vi "HART.vi"(4 "Error In":errorcluster, 7 "Command":string) -> (0 "Error Out":errorcluster, 3 "Response":string)   [LabVIEW 2018]
uses:
  MOKO_LabViewLibrary/MokoLowLevel/MokoLowLovelControl/MLLC_ConnectCluster.ctl
  MOKO_LabViewLibrary/MokoLowLevel/MokoLowLovelControl/MLLC_InterfaceType.ctl
  MOKO_LabViewLibrary/MokoLowLevel/MokoLowLovelControl/MLLC_OpenedSession.ctl
  MOKO_LabViewLibrary/MokoLowLevel/MokoLowLovelControl/MLLC_InterfaceSettings.ctl
  MOKO_LabViewLibrary/MokoLowLevel/MokoLowLovelControl/MLLC_InterfaceKind.ctl
panel:
  in  "Settings":T6={"Saved Data"=variant, "Permanent data"={"Connect"={"InterfaceType"=enum."VISA", "OpenedSession"="", "InterfaceSettings"={"Interface"=enum."RS232", "EOS 4 read"=enum."LF (\\n)", "EOS 4 write"=enum."LF (\\n)", "TMO, ms"=10000, "Sett"=variant(cluster{"Baud Rate":u32, "Data Bits":u16, "Parity":u16, "Stop Bits":u16, "Flow Control":u16, "Eho":bool} {"Baud Rate"=75, "Data Bits"=0, "Parity"=0, "Stop Bits"=0, "Flow Control"=0, "Eho"=FALSE})}}, "Value"={"I"=0.0, "P"=0.0, "T"=0.0}, "String"="empty"}}
  in  "Error Code":u32
  in  "Driver Name":string="HART"
  in  "Mode":T7(ring)=enum."Check"
  # "HART"
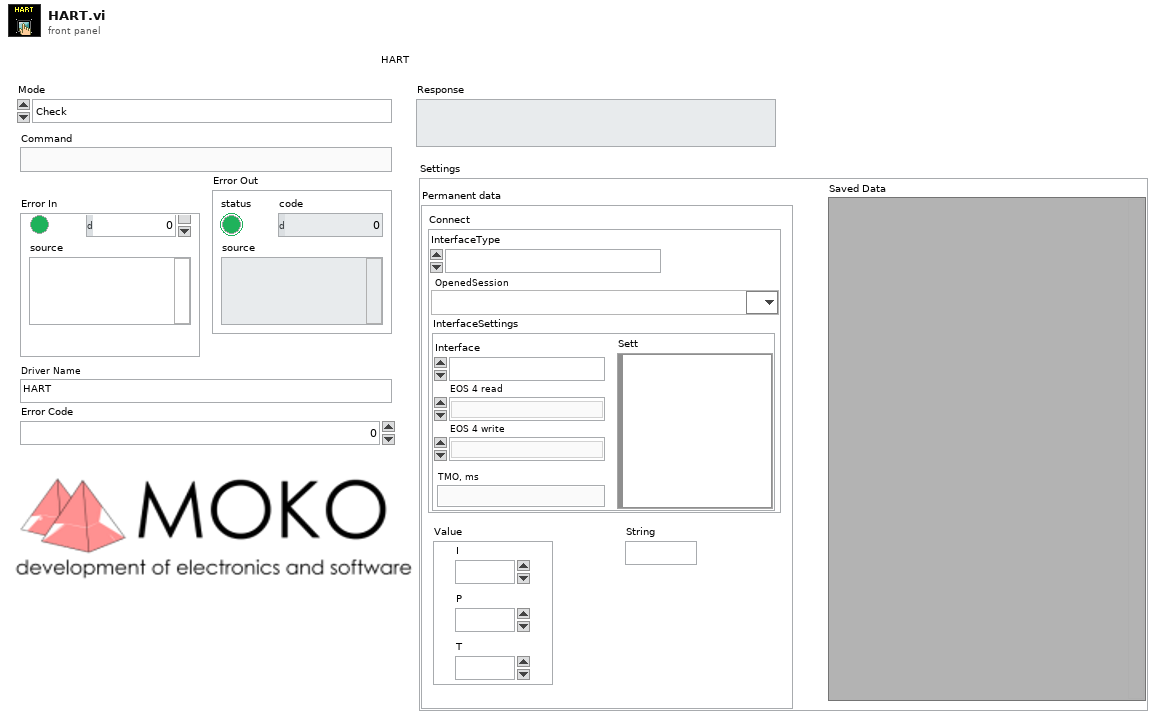
[diagram p1: front panel]
types:
  T1 = typedef "MLLC_ConnectCluster.ctl" = cluster{"InterfaceType":T2, "OpenedSession":T3, "InterfaceSettings":T4}
  T2 = typedef "MLLC_InterfaceType.ctl" = enum16{"VISA", "Prologix USB-GPIB"}
  T3 = typedef "MLLC_OpenedSession.ctl" = refnum<visa-resource-name>
  T4 = typedef "MLLC_InterfaceSettings.ctl" = cluster{"Interface":T5, "EOS 4 read":enum16{"Default (=EOS 4 write)", "CR (\\r)", "LF (\\n)", "None"}, "EOS 4 write":enum16{"CR+LF (\\r\\n)", "CR (\\r)", "LF (\\n)", "None"}, "TMO, ms":i32, "Sett":variant}
  T5 = typedef "MLLC_InterfaceKind.ctl" = enum16{"RS232", "GPIB", "USB", "Ethernet", "another"}
  T6 = cluster{"Saved Data":variant, "Permanent data":cluster{"Connect":T1, "Value":cluster{"I":dbl, "P":dbl, "T":dbl}, "String":string}}
  T7 = enum16{"get", "set", "close", "Init", "Check", "ID"}
  T8 = cluster{"Connect":T1, "Value":cluster{"I":dbl, "P":dbl, "T":dbl}, "String":string}
  T9 = typedef "MLLC_Mode.ctl" = enum16{"get", "set", "close", "Init", "Check"}
  T10 = typedef "MLLC_Error.ctl" = errorcluster
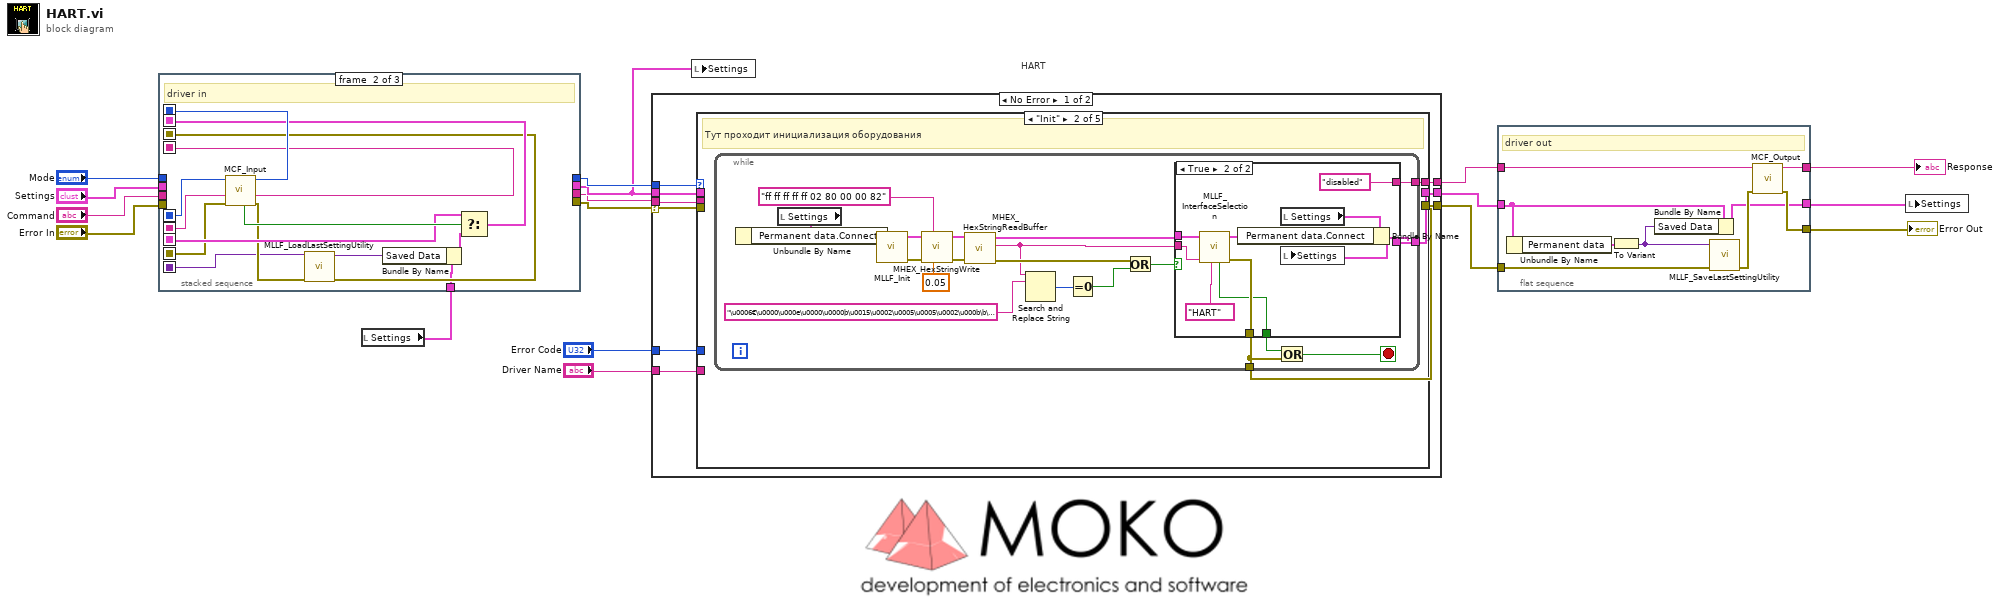
[diagram p0: block diagram]
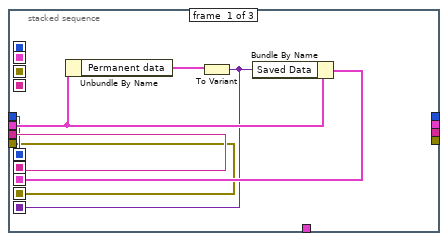
[diagram p2: hidden frame]
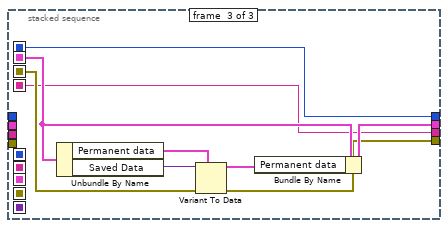
[diagram p3: hidden frame]
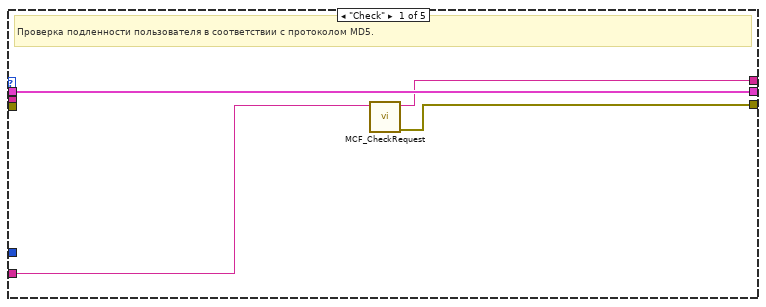
[diagram p4: hidden frame]
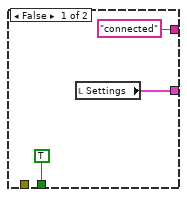
[diagram p5: hidden frame]
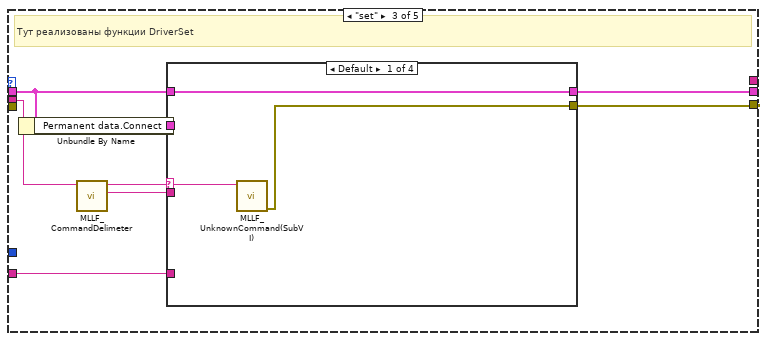
[diagram p6: hidden frame]
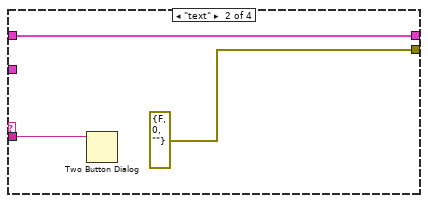
[diagram p7: hidden frame]
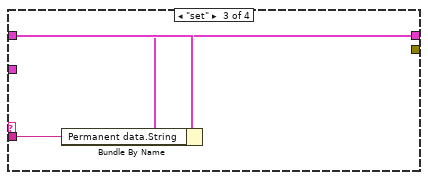
[diagram p8: hidden frame]
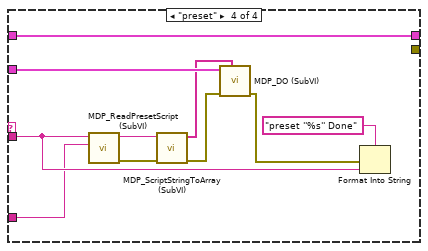
[diagram p9: hidden frame]
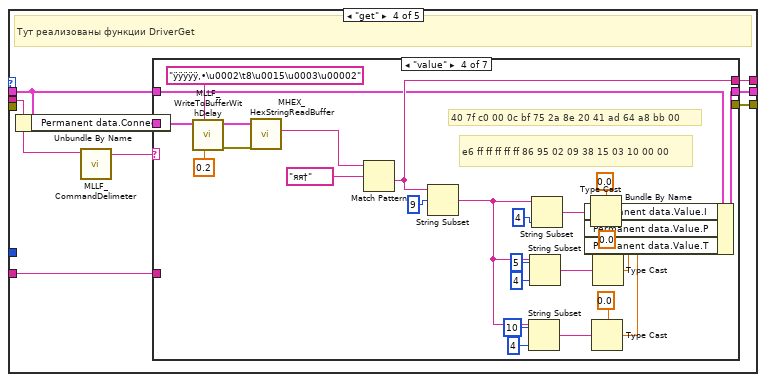
[diagram p10: hidden frame]
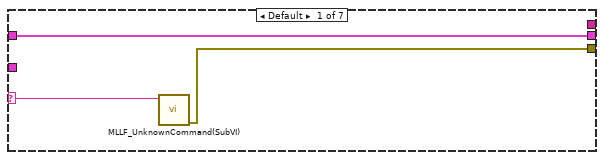
[diagram p11: hidden frame]
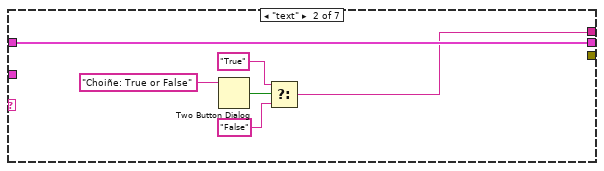
[diagram p12: hidden frame]
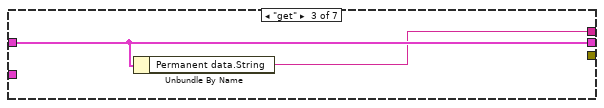
[diagram p13: hidden frame]
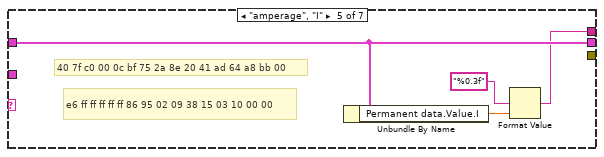
[diagram p14: hidden frame]
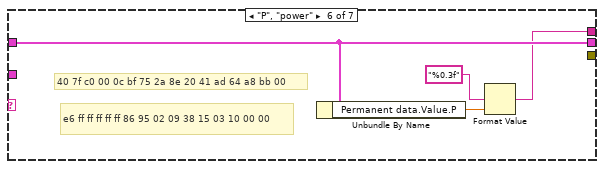
[diagram p15: hidden frame]
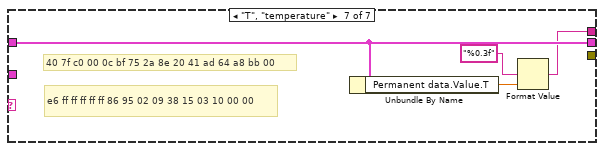
[diagram p16: hidden frame]
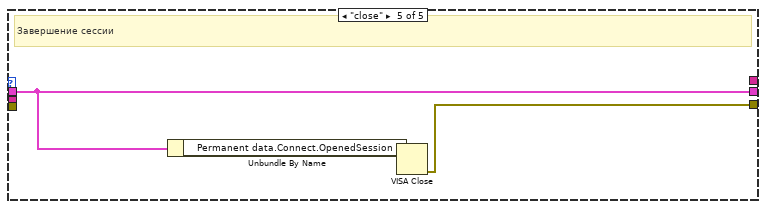
[diagram p17: hidden frame]
diagram:
  # "HART"
  n1 = local read "Settings"() -> (w13:T6)
  n2 = stacked-sequence {
    seq-local: [w20 _ _] -> [_ w36 _]
    seq-local: [w19 _ _] -> [_ w37 _]
    seq-local: [w22 _ _] -> [_ w32 _]
    seq-local: [w18 _ _] -> [_ w31 _]
    seq-local: [w21 _ _] -> [_ w27 _]
    seq-local: [_ w28 _] -> [_ _ w44]
    seq-local: [_ w38 _] -> [_ _ w41]
    seq-local: [_ w35 _] -> [_ _ w40]
    seq-local: [_ w34 _] -> [_ _ w45]
    tunnel: "Command" -> [w20 _ _]
    tunnel: "Mode" -> [w19 _ _]
    tunnel: "Error In" -> [w18 _ _]
    tunnel: "Settings" -> [w23 _ _]
    tunnel: w13 -> [_ w26 _]
    tunnel: [_ _ w40] -> w12
    tunnel: [_ _ w43] -> w14
    tunnel: [_ _ w42] -> w11
    tunnel: [_ _ w41] -> w15
    frame #0 {
      n3 = Unbundle By Name(w23) -> ("Permanent data"=w24:T8)
      n4 = To Variant(anything=w24) -> (Variant=w21:variant)
      n5 = Bundle By Name(cluster=w23, "Saved Data"=w21) -> (w22:T6)
    }
    frame #1 {
      # "driver in"
      n6 = call "MCF_Input.vi"("Error In"=w31, "Command in"=w36, "Mode in"=w37) -> ("Error Out"=w30:errorcluster, "Command out"=w35:string, "Mode out"=w38:T9, "Boolean"=w33:bool)  [unwired: 5 in]
      n7 = call "MLLF_LoadLastSettingUtility.vi"("Error In"=w30, "Save data in"=w27) -> ("Error Out"=w28:errorcluster, "Save data out"=w25:variant)  [unwired: 8 in]
      n8 = Bundle By Name(cluster=w26, "Saved Data"=w25) -> (w29:T6)
      n9 = Select(t=w32, s=w33, f=w29) -> (s? t:f=w34:T6)
    }
    frame #2 {
      n10 = Unbundle By Name(w45) -> ("Permanent data"=w46:T8, "Saved Data"=w39:variant)
      n11 = Variant To Data(error in=w44, type=w46, Variant=w39) -> (data=w47:T8, error out=w42:errorcluster)
      n12 = Bundle By Name(cluster=w45, "Permanent data"=w47) -> (w43:T6)
    }
  }
  n13 = case shown="No Error" w11 {
    selector: w11 -> [w53 w184]
    tunnel: [w48 w184] -> w4
    tunnel: w15 -> [w56 _]
    tunnel: [w55 _] -> w6
    tunnel: w12 -> [w54 _]
    tunnel: w14 -> [w50 w183]
    tunnel: "Error Code" -> [w52 _]
    tunnel: "Driver Name" -> [w51 _]
    tunnel: [w49 w183] -> w5
    frame No Error {
      n14 = case shown="\"Init\"" w56 {
        tunnel: [w58 w62 _ w124 _] -> w55
        tunnel: w54 -> [_ _ w99 w127 _]
        tunnel: w53 -> [_ _ _ _ _]
        tunnel: w52 -> [_ _ _ _ _]
        tunnel: w51 -> [w59 _ w101 w125 _]
        tunnel: w50 -> [w60 _ w103 w130 w181]
        tunnel: [w60 w63 w102 w129 w181] -> w49
        tunnel: [w57 w61 w96 w123 w180] -> w48
        frame "Check" {
          # "Проверка подленности пользователя в соответствии с протоколом MD5."
          n15 = call "MCF_CheckRequest.vi"("Driver Name"=w59) -> ("Error Out"=w57:errorcluster, "Output String"=w58:string)  [unwired: 9 in]
        }
        frame "Init" {
          # "Тут проходит инициализация оборудования"
          n16 = while {
            tunnel: [w80] -> w63
            tunnel: [w78] -> w62
            tunnel: [w65] -> w61
            stop <- w82 stop-if-true
            n17 = local read "Settings"() -> (w81:T6)
            n18 = Unbundle By Name(w81) -> ("Permanent data.Connect"=w79:T1)
            n19 = call "MLLF_Init.vi"("DriverConnect in"=w79) -> ("Error Out"=w75:errorcluster, "DriverConnect out"=w76:T1)  [unwired: 7 in]
            n20 = call "MHEX_HexStringWrite.vi"("Delay Time (s)"=0.05, "Command"="ff ff ff ff ff 02 80 00 00 82" ("commands"), "error in"=w75, "DriverConnect in"=w76) -> ("error out"=w73:T10, "DriverConnect out"=w74:T1)  [unwired: 6 in]
            n21 = call "MHEX_HexStringReadBuffer.vi"("error in"=w73, "DriverConnect in"=w74) -> ("error out"=w68:T10, "String from device out"=w64:string, "DriverConnect out"=w72:T1)  [unwired: 6 in, 1 out]
            n22 = Search and Replace String(input string=w64, search string="\u0006€\u0000\u000e\u0000\u0000þ\u0015\u0002\u0005\u0005\u0002\u000b\b\u0000\t8\u0015D\u0000") -> (number of replacements=w70:i32)  [unwired: 6 in, 3 out]
            n23 = Equal To 0?(x=w70) -> (x = 0?=w69:bool)
            n24 = Or(x=w68, y=w69) -> (x .or. y?=w67:bool)
            n25 = case shown="True" w67 {
              tunnel: w72 -> [_ w94]
              tunnel: [TRUE w89] -> w83
              tunnel: [_ w95] -> w65
              tunnel: [w85 w90] -> w80
              tunnel: ["connected" "disabled"] -> w78
              tunnel: w64 -> [_ w87]
              frame False {
                n26 = local read "Settings"() -> (w85:T6)
              }
              frame True {
                n27 = call "MLLF_InterfaceSelection.vi"("Driver Name"="HART" ("String"), "Answer:"=w87, "DriverConnect in"=w94) -> ("error out"=w95:T10, "DriverConnect out"=w92:T1, "stop init?"=w89:bool)  [unwired: 4 in, 2 out]
                n28 = local read "Settings"() -> (w91:T6)
                n29 = Bundle By Name(cluster=w91, "Permanent data.Connect"=w92) -> (w90:T6)
                n30 = local write "Settings"(w90) -> ()
              }
            }
            n31 = Or(x=w83, y=w65) -> (x .or. y?=w82:bool)
          }
        }
        frame "set" {
          # "Тут реализованы функции DriverSet"
          n32 = Unbundle By Name(w103) -> ("Permanent data.Connect"=w100:T1)
          n33 = call "MLLF_CommandDelimeter.vi"("command with param"=w99) -> ("param 1"=w97:string, "command"=w98:string)  [unwired: 6 in, 3 out]
          n34 = case shown="Default" w98 {
            selector: w98 -> [w105 _ _ _]
            tunnel: [w106 w109 w111 w113] -> w102
            tunnel: w103 -> [w106 w109 w112 w113]
            tunnel: w100 -> [_ _ _ w117]
            tunnel: w97 -> [_ w107 w110 w116]
            tunnel: [w104 errorcluster {"status"=FALSE, "code"=0, "source"=""} ("error IO") _ _] -> w96
            tunnel: w101 -> [_ _ _ w115]
            frame Default {
              n35 = call "MLLF_UnknownCommand(SubVI).vi"("Unknown command"=w105) -> ("error out"=w104:errorcluster)  [unwired: 10 in]
            }
            frame "text" {
              n36 = Two Button Dialog(message=w107) -> ()  [unwired: 2 in, 1 out]
            }
            frame "set" {
              n37 = Bundle By Name(cluster=w112, "Permanent data.String"=w110) -> (w111:T6)
            }
            frame "preset" {
              n38 = call "MDP_ReadPresetScript (SubVI).vi"("Driver Name"=w115, "String in"=w116) -> ("Error Out"=w120:errorcluster, "String out"=w121:string)  [unwired: 8 in]
              n39 = call "MDP_ScriptStringToArray (SubVI).vi"("Error In"=w120, "String script"=w121) -> ("Error Out"=w122:errorcluster, "Array script"=w114:string[])  [unwired: 8 in]
              n40 = call "MDP_DO (SubVI).vi"("Array script"=w114, "Error in (no error)"=w122, "DriverConnect in"=w117) -> ("Error Out"=w118:errorcluster)  [unwired: 7 in, 1 out]
              n41 = Format Into String(format string="preset ''%s'' Done" ("Befor substring"), error in=w118, w116) -> ()  [unwired: 1 in, 2 out]
            }
          }
        }
        frame "get" {
          # "Тут реализованы функции DriverGet"
          n42 = Unbundle By Name(w130) -> ("Permanent data.Connect"=w128:T1)
          n43 = call "MLLF_CommandDelimeter.vi"("command with param"=w127) -> ("command"=w126:string)  [unwired: 6 in, 4 out]
          n44 = case shown="\"value\"" w126 {
            selector: w126 -> [w132 _ _ _ _ _ _]
            tunnel: w128 -> [_ _ _ w166 _ _ _]
            tunnel: w130 -> [w133 w139 w141 w147 w171 w175 w179]
            tunnel: [w133 w139 w141 w143 w171 w175 w179] -> w129
            tunnel: [_ w134 w140 w161 w168 w172 w176] -> w124
            tunnel: [w131 _ _ _ _ _ _] -> w123
            tunnel: w125 -> [_ _ _ _ _ _ _]
            frame Default {
              n45 = call "MLLF_UnknownCommand(SubVI).vi"("Unknown command"=w132) -> ("error out"=w131:errorcluster)  [unwired: 10 in]
            }
            frame "text" {
              n46 = Two Button Dialog(message="Choiñe: True or False") -> (T button?=w138:bool)  [unwired: 2 in]
              n47 = Select(t="True" ("string"), s=w138, f="False" ("string")) -> (s? t:f=w134:string)
            }
            frame "get" {
              n48 = Unbundle By Name(w141) -> ("Permanent data.String"=w140:string)
            }
            frame "value" {
              # "40 7f c0 00 0c bf 75 2a 8e 20 41 ad 64 a8 bb 00"
              # "e6 ff ff ff ff ff 86 95 02 09 38 15 03 10 00 00"
              n49 = call "MLLF_WriteToBufferWithDelay.vi"("Delay Time ( 0,05 s)"=0.2 ("Delay Time (s)"), "Command"="ÿÿÿÿÿ‚•\u0002\t8\u0015\u0003\u00002", "DriverConnect in"=w166) -> ("Error Out"=w164:errorcluster, "DriverConnect out"=w165:T1)  [unwired: 7 in]
              n50 = call "MHEX_HexStringReadBuffer.vi"("error in"=w164, "DriverConnect in"=w165) -> ("String from device out"=w142:string)  [unwired: 6 in, 3 out]
              n51 = Match Pattern(string=w142, regular expression="яя†" ("HEX Response")) -> (after substring=w161:string)  [unwired: 1 in, 3 out]
              n52 = String Subset(string=w161, offset (0)=9) -> (substring=w149:string)  [unwired: 1 in]
              n53 = String Subset(string=w149, offset (0)=10, length (rest)=4 ("offset (0)")) -> (substring=w148:string)
              n54 = String Subset(string=w149, offset (0)=5, length (rest)=4 ("offset (0)")) -> (substring=w154:string)
              n55 = String Subset(string=w149, length (rest)=4 ("offset (0)")) -> (substring=w157:string)  [unwired: 1 in]
              n56 = Type Cast(type=sgl 0.0, x=w157) -> (*(type *) &x=w146:sgl)
              n57 = Type Cast(type=sgl 0.0, x=w148) -> (*(type *) &x=w144:sgl)
              n58 = Type Cast(type=sgl 0.0, x=w154) -> (*(type *) &x=w145:sgl)
              n59 = Bundle By Name(cluster=w147, "Permanent data.Value.I"=w146, "Permanent data.Value.P"=w145, "Permanent data.Value.T"=w144) -> (w143:T6)
            }
            frame "amperage", "I" {
              # "40 7f c0 00 0c bf 75 2a 8e 20 41 ad 64 a8 bb 00"
              # "e6 ff ff ff ff ff 86 95 02 09 38 15 03 10 00 00"
              n60 = Unbundle By Name(w171) -> ("Permanent data.Value.I"=w170:dbl)
              n61 = Format Value(format string="%0.3f", value (0)=w170) -> (output string=w168:string)  [unwired: 1 in]
            }
            frame "P", "power" {
              # "40 7f c0 00 0c bf 75 2a 8e 20 41 ad 64 a8 bb 00"
              # "e6 ff ff ff ff ff 86 95 02 09 38 15 03 10 00 00"
              n62 = Unbundle By Name(w175) -> ("Permanent data.Value.P"=w174:dbl)
              n63 = Format Value(format string="%0.3f", value (0)=w174) -> (output string=w172:string)  [unwired: 1 in]
            }
            frame "T", "temperature" {
              # "40 7f c0 00 0c bf 75 2a 8e 20 41 ad 64 a8 bb 00"
              # "e6 ff ff ff ff ff 86 95 02 09 38 15 03 10 00 00"
              n64 = Unbundle By Name(w179) -> ("Permanent data.Value.T"=w178:dbl)
              n65 = Format Value(format string="%0.3f", value (0)=w178) -> (output string=w176:string)  [unwired: 1 in]
            }
          }
        }
        frame "close" {
          # "Завершение сессии"
          n66 = Unbundle By Name(w181) -> ("Permanent data.Connect.OpenedSession"=w182:T3)
          n67 = VISA Close(VISA resource name=w182) -> (error out=w180:errorcluster)  [unwired: 1 in]
        }
      }
    }
    frame Error {
    }
  }
  n68 = local write "Settings"(w14) -> ()
  n69 = flat-sequence {
    tunnel: [w193] -> w3
    tunnel: [w192] -> w1
    tunnel: w6 -> [w191]
    tunnel: w4 -> [w190]
    tunnel: w5 -> [w186]
    tunnel: [w188] -> w2
    frame #0 {
      # "driver out"
      n70 = Unbundle By Name(w186) -> ("Permanent data"=w185:T8)
      n71 = To Variant(anything=w185) -> (Variant=w187:variant)
      n72 = Bundle By Name(cluster=w186, "Saved Data"=w187) -> (w188:T6)
      n73 = call "MLLF_SaveLastSettingUtility.vi"("error in"=w190, "Saved Data"=w187) -> ("error out"=w189:T10)  [unwired: 8 in, 1 out]
      n74 = call "MCF_Output.vi"("Error In"=w189, "Input"=w191) -> ("Error Out"=w192:errorcluster, "Output"=w193:string)  [unwired: 8 in]
    }
  }
  n75 = local write "Settings"(w2) -> ()
  "Response" <- w3
  "Error Out" <- w1
